vi "Speed2Power.vi"() -> ()   [LabVIEW 2017]
panel:
  out "Power":dbl format="%#_13g"
  in  "Speed":dbl format="%#_13g"
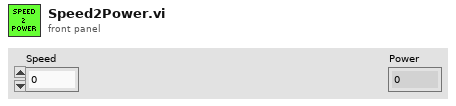
[diagram p1: front panel]
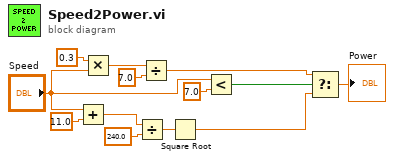
[diagram p0: block diagram]
diagram:
  n1 = Add(x="Speed", y=11.0) -> (x+y=w3:dbl)
  n2 = Multiply(x=0.3, y="Speed") -> (x*y=w10:dbl)
  n3 = Divide(x=w3, y=240.0) -> (x/y=w2:dbl)
  n4 = Divide(x=w10, y=7.0) -> (x/y=w8:dbl)
  n5 = Square Root(x=w2) -> (sqrt(x)=w1:dbl)
  n6 = Less?(x="Speed", y=7.0) -> (x < y?=w12:bool)
  n7 = Select(t=w8, s=w12, f=w1) -> (s? t:f=→"Power":dbl)
